vi "Use Case4.vi"() -> ()   [LabVIEW 2021, in "uCanDriver.lvlib" / "uCAN.lvclass"]
uses:
  uCAN.lvclass
  typedefs/frame.ctl
  typedefs/bitrates.ctl
panel:
  in  "Trace length":u64=100
  out "Table Control":string[][](table)
  in  "New Frame":T1
  in  "Bitrates":T2=enum."500 kbit/s"
  in  "COM port":refnum<visa-resource-name>="COM9"
  in  "Transmit Frame":bool
  in  "stop":bool
  out "Received Frames":T1[](array[typedef]) {"Data" format="%.0x"}
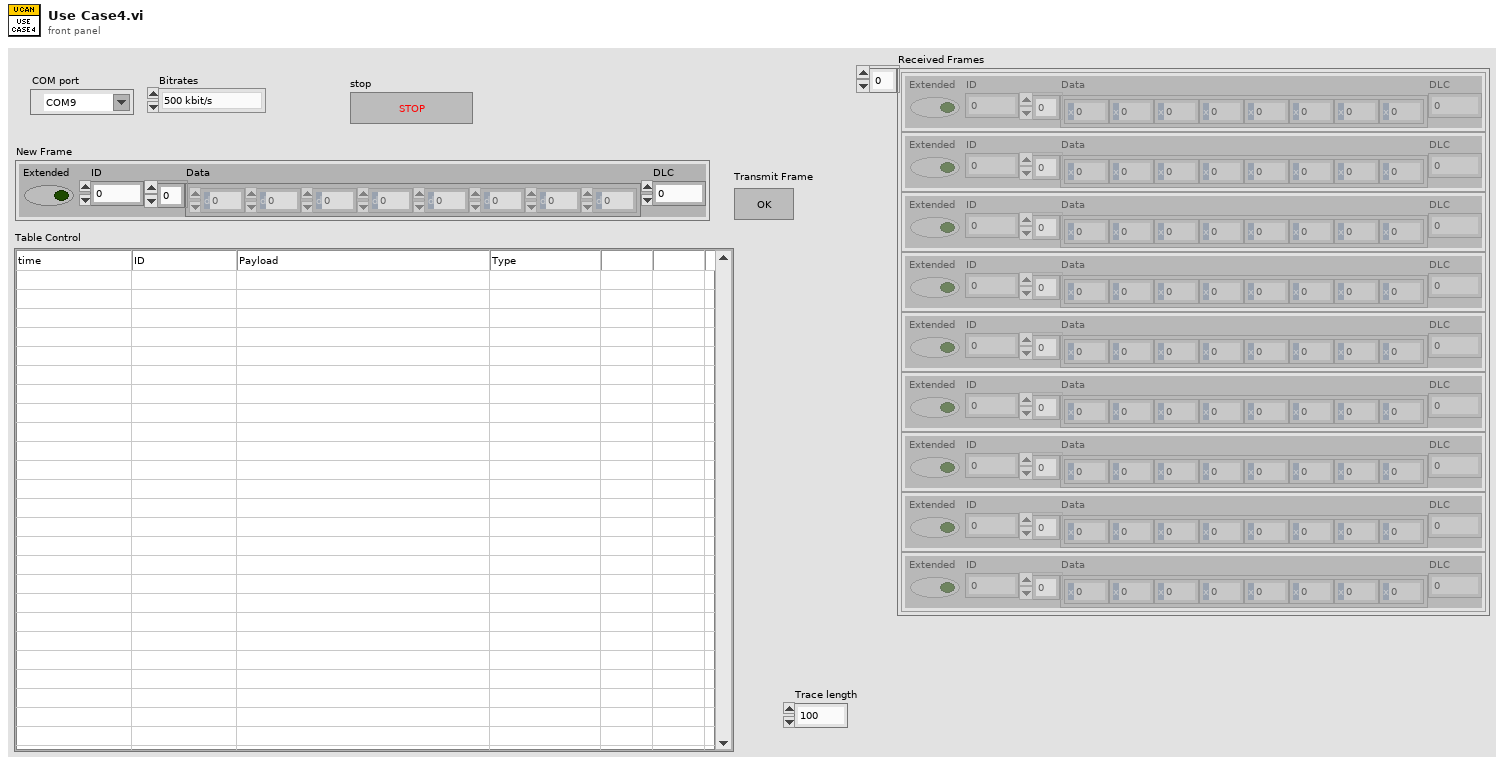
[diagram p1: front panel]
types:
  T1 = typedef "uCanDriver.lvlib/uCAN.lvclass/frame.ctl" = cluster{"Extended":bool, "ID":u32, "Data":u8[], "DLC":u8}
  T2 = typedef "uCanDriver.lvlib/uCAN.lvclass/bitrates.ctl" = enum16{"100 kbit/s", "125 kbit/s", "250 kbit/s", "500 kbit/s", "800 kbit/s", "1 Mbit/s"}
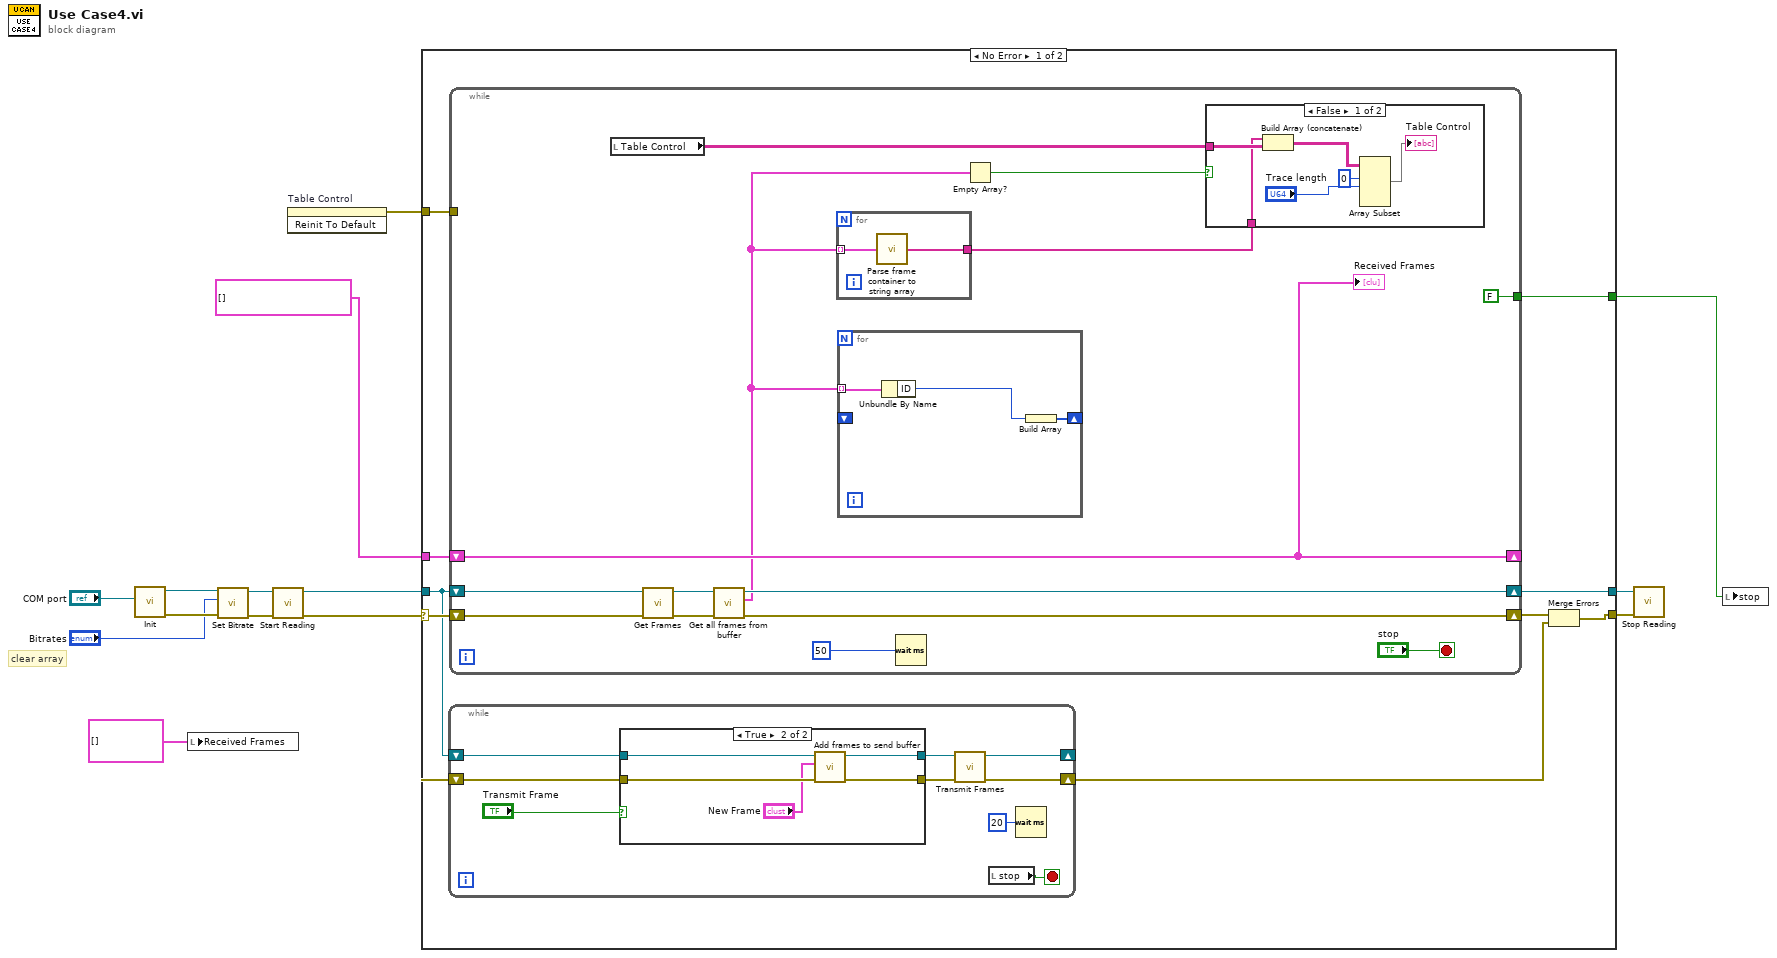
[diagram p0: block diagram]
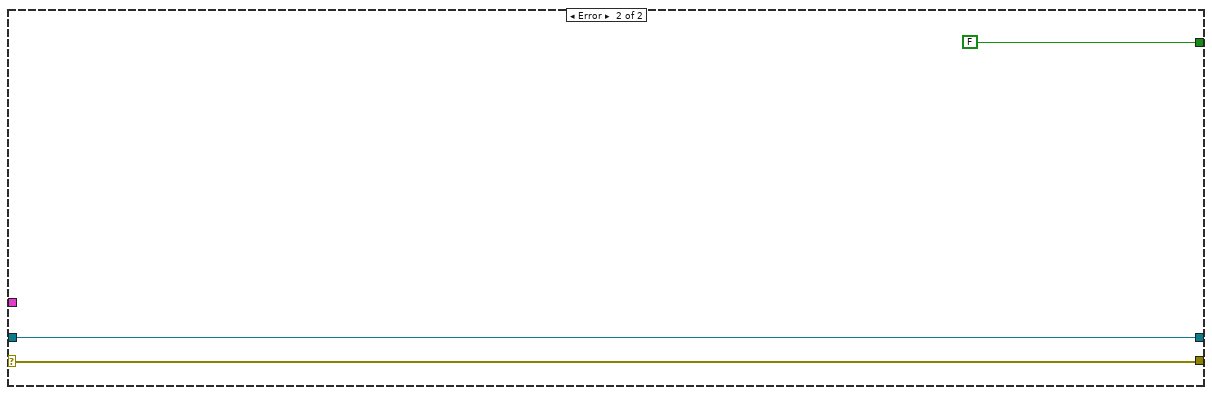
[diagram p4: hidden frame]
diagram:
  # "clear array"
  n1 = call "Init.vi"("COM port"="COM port") -> ("error out"=w12:errorcluster, "uCAN out"=w13:refnum<class "uCAN.lvclass">)  [unwired: 9 in]
  n2 = local write "Received Frames"(T1[] [] ("Received Frames Array")) -> ()
  n3 = call "Set Bitrate.vi"("error in (no error)"=w12, "Bitrates"="Bitrates", "uCAN in"=w13) -> ("error out"=w7:errorcluster, "uCAN out"=w5:refnum<class "uCAN.lvclass">)  [unwired: 7 in]
  n4 = call "Start Reading.vi"("error in (no error)"=w7, "uCAN in"=w5) -> ("error out"=w6:errorcluster, "uCAN out"=w4:refnum<class "uCAN.lvclass">)  [unwired: 8 in]
  n5 = invoke on="Table Control" class="Tbl (strict)" method="Reinit To Default"() -> (error out=w3:errorcluster)  [unwired: 3 in, 2 out]
  n6 = case shown="No Error" w6 {
    selector: w6 -> [w19 w67]
    tunnel: [w23 w66] -> w10
    tunnel: [w21 w67] -> w8
    tunnel: w4 -> [w18 w66]
    tunnel: w3 -> [w17 _]
    tunnel: [w16 FALSE ("stop")] -> w2
    tunnel: T1[] [] ("Received Frames") -> [w15 _]
    frame No Error {
      n7 = while {
        shift-right: [w51] -> _
        shift-left: w18 -> [w57]
        shift-right: [w53] -> w20
        shift-left: w19 -> [w56]
        stop <- w50 stop-if-true
        n8 = case shown="True" "Transmit Frame" {
          tunnel: w57 -> [w59 w64]
          tunnel: w56 -> [w58 w63]
          tunnel: [w58 w62] -> w55
          tunnel: [w59 w61] -> w52
          frame False {
          }
          frame True {
            n9 = call "Add frames to send buffer.vi"("error in (no error)"=w63, "New Frame"="New Frame", "uCAN in"=w64) -> ("error out"=w62:errorcluster, "uCAN out"=w61:refnum<class "uCAN.lvclass">)  [unwired: 7 in]
          }
        }
        n10 = call "Transmit Frames.vi"("error in (no error)"=w55, "uCAN in"=w52) -> ("error out"=w53:errorcluster, "uCAN out"=w51:refnum<class "uCAN.lvclass">)  [unwired: 8 in]
        n11 = local read "stop"() -> (w50:bool)
        n12 = Wait (ms)(milliseconds to wait=u32 20) -> ()  [unwired: 1 out]
      }
      n13 = while {
        shift-right: [w33] -> w23
        shift-left: w18 -> [w37]
        shift-right: [w32] -> w22
        shift-left: w19 -> [w36]
        tunnel: w17 -> [_]
        tunnel: [FALSE ("stop")] -> w16
        shift-right: [w25] -> _
        shift-left: w15 -> [w25]
        stop <- "stop" stop-if-true
        n14 = local read "Table Control"() -> (w29:string[][])
        n15 = call "Get Frames.vi"("error in (no error)"=w36, "uCAN in"=w37) -> ("error out"=w35:errorcluster, "uCAN out"=w34:refnum<class "uCAN.lvclass">)  [unwired: 7 in, 1 out]
        n16 = call "Get all frames from buffer.vi"("error in (no error)"=w35, "uCAN in"=w34) -> ("error out"=w32:errorcluster, "Received Frames Array"=w24:T1[], "uCAN out"=w33:refnum<class "uCAN.lvclass">)  [unwired: 7 in]
        n17 = for {
          tunnel: [w42] -> w26
          tunnel: w24 -> [w41] mode=indexing
          n18 = call "Parse frame container to string array.vi"("Frame"=w41) -> ("String array"=w42:string[])
        }
        n19 = for {
          tunnel: w24 -> [w40] mode=indexing
          shift-right: [w38] -> _
          shift-left: _ -> [_]
          n20 = Unbundle By Name(w40) -> ("ID"=w39:u32)
          n21 = Build Array(w39) -> (w38:u32[])
        }
        n22 = Wait (ms)(milliseconds to wait=u32 50) -> ()  [unwired: 1 out]
        n23 = Empty Array?(array=w24) -> (empty?=w28:bool)
        n24 = case shown="False" w28 {
          tunnel: w29 -> [w48 _]
          tunnel: w26 -> [w47 _]
          frame False {
            n25 = Build Array (concatenate)(w47, w48) -> (w44:string[][])
            n26 = Array Subset(array=w44, index (row)=0 ("index"), length (row)="Trace length") -> (→"Table Control":string[][])  [unwired: 2 in]
          }
          frame True {
          }
        }
        "Received Frames" <- w25
      }
      n27 = Merge Errors(w22, w20) -> (w21:errorcluster)
    }
    frame Error {
    }
  }
  n28 = call "Stop Reading.vi"("error in (no error)"=w8, "uCAN in"=w10) -> ()  [unwired: 8 in, 2 out]
  n29 = local write "stop"(w2) -> ()
